vi "Read Element of conversion_unit.vi"(8 "error in (no error)":errorcluster, 10 "axis":i32, 11 "DLOwis in":refnum<class "DLOwis.lvclass">) -> (0 "error out":errorcluster, 2 "Numeric":dbl, 3 "DLOwis out":refnum<class "DLOwis.lvclass">)   [LabVIEW 2019, in "DLOwis.lvclass"]
uses:
  DLOwis.lvclass
  DLOwis.lvclass/DLOwis.ctl
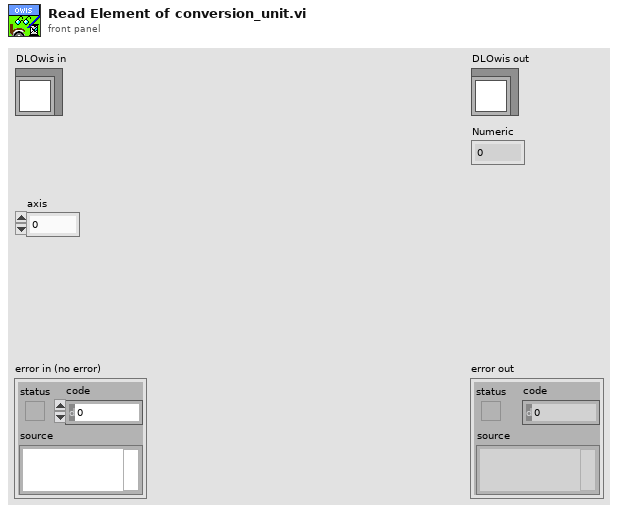
[diagram p1: front panel]
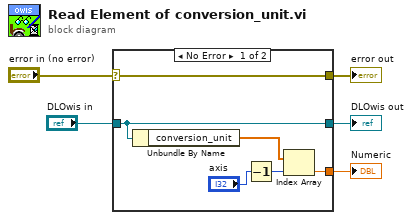
[diagram p0: block diagram]
diagram:
  n1 = case shown="No Error" "error in (no error)" {
    selector: "error in (no error)" -> [w11 w12]
    tunnel: [w11 w12] -> w4
    tunnel: [w10 w13] -> w2
    tunnel: "DLOwis in" -> [w10 w13]
    tunnel: [w7 _] -> w1
    frame No Error {
      n2 = Unbundle By Name(w10) -> ("conversion_unit"=w9:dbl[])
      n3 = Decrement(x="axis") -> (x-1=w6:i32)
      n4 = Index Array(array=w9, index=w6) -> (element=w7:dbl)
    }
    frame Error {
    }
  }
  "error out" <- w4
  "DLOwis out" <- w2
  "Numeric" <- w1
